vi "TestBed.vi"() -> ()   [LabVIEW 2017]
uses:
  <vilib>/gpm_packages/@cs/Network-sink/Source/Network Interface/Network Interface/Network Interface.lvclass
  f39cf365-6f17-4216-9592-3f82a383dcb0.vi
  <vilib>/gpm_packages/@cs/Network-sink/Source/HeaderMessageProtocol/HeaderMessageProtocol.lvclass
  <vilib>/gpm_packages/@cs/event-logger/Source/String Control Sink/String Control Sink.lvclass
  <vilib>/gpm_packages/@cs/event-logger/Source/Composed Log/Types/Log Level.ctl
  <vilib>/gpm_packages/@cs/event-logger/Source/Composed Log/Composed Log.lvlib
  <vilib>/gpm_packages/@cs/event-logger/Source/Composed Log/LoggerReference/LoggerReference.lvclass
  86a66f69-750b-45a4-9a60-f207d6d0df32.vi
  <vilib>/gpm_packages/@cs/Network-sink/Source/Network Interface/IConnectionFactory/IConnectionFactory.lvclass
  <vilib>/gpm_packages/@cs/Network-sink/Source/Network Interface/IMessagingProtocol/IMessagingProtocol.lvclass
panel:
  out "Array":string[](array[string])
  out "String":string
  out "Numeric 2":dbl
  out "Numeric":dbl
  out "error out":errorcluster
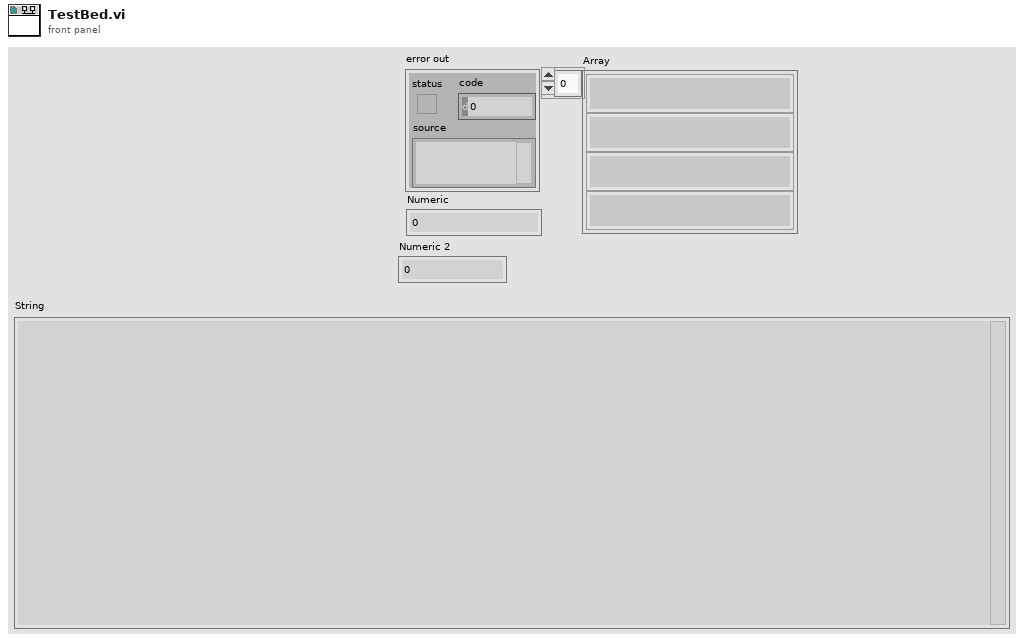
[diagram p1: front panel]
types:
  T1 = typedef "Composed Log.lvlib/Log Level.ctl" = enum16{"Debug", "Info", "Warning", "Error", "Critical"}
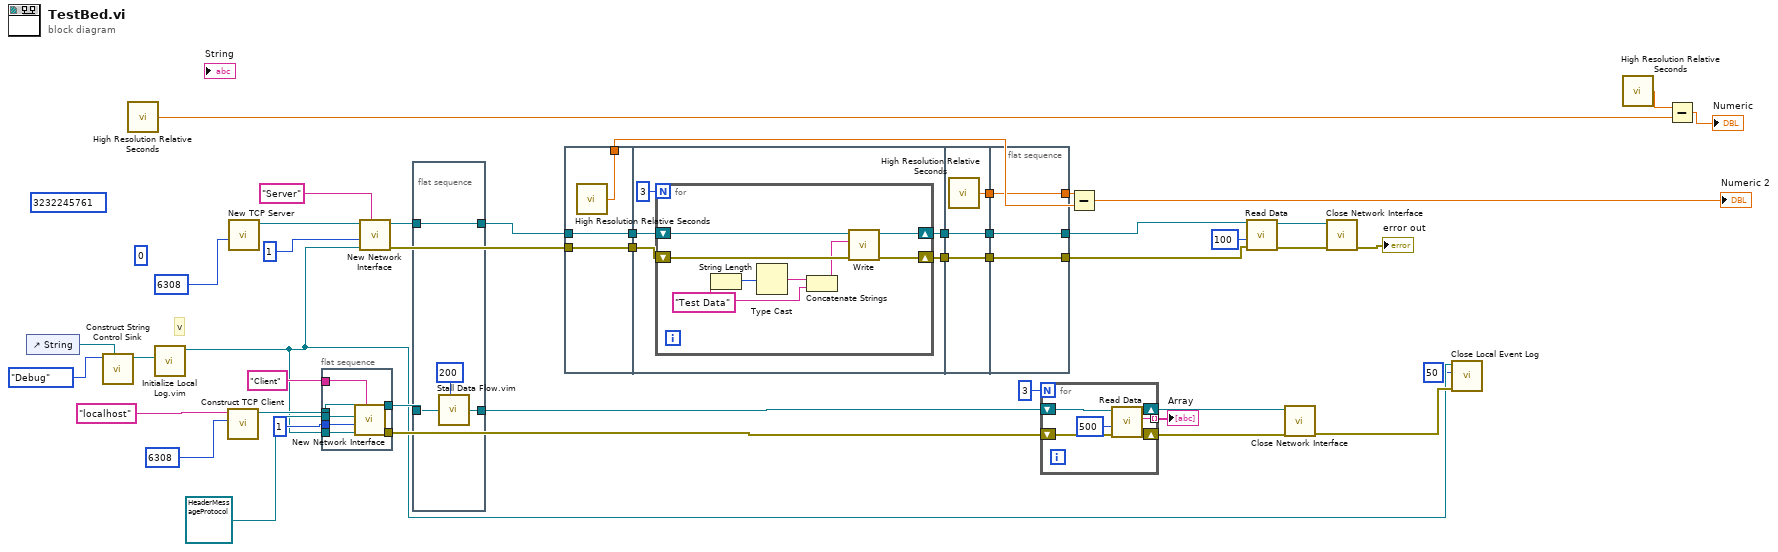
[diagram p0: block diagram]
diagram:
  (unwired) u32 3232245761
  (unwired) u32 0 ("net address")
  # "v"
  n1 = control-ref of="String"() -> (w11:refnum<vi>)
  n2 = call <vilib>:"Construct String Control Sink.vi"("Str Refnum"=w11, "LogLevel"=Log_Level."Debug") -> ("String Control Sink out"=w9:refnum<class "String Control Sink.lvclass">)  [unwired: 9 in]
  n3 = call <vilib>:"High Resolution Relative Seconds.vi"() -> ("relative seconds"=w44:dbl)
  n4 = call "Initialize Local Log.vim"("Startup Sink(s)"=w9) -> ("Log Instance Reference"=w5:refnum<class "LoggerReference.lvclass">)  [unwired: 8 in, 2 out]
  n5 = call <vilib>:"Construct TCP Client.vi"("Remote Port or Service Name"=u16 6308 ("Port"), "Address"="localhost") -> ("TCP Client out"=w39:refnum<class "TCP Client.lvclass">)  [unwired: 9 in]
  n6 = call <vilib>:"New TCP Server.vi"("Port"=u16 6308) -> ("TCP Server out"=w37:refnum<class "TCP Server.lvclass">)  [unwired: 10 in]
  n7 = flat-sequence {
    tunnel: w39 -> [w52]
    tunnel: [w51] -> w29
    tunnel: [w50] -> w24
    tunnel: refnum<class "HeaderMessageProtocol.lvclass"> refnum ("Network Sink.lvlib:HeaderMessageProtocol.lvclass") -> [w49]
    tunnel: 1 ("Max Number of Connections") -> [w48]
    tunnel: "Client" ("Log Alias") -> [w47]
    tunnel: w5 -> [w46]
    frame #0 {
      n8 = call <vilib>:"New Network Interface.vi"("Log Alias"=w47, "Log Instance"=w46, "Max Number of Connections to Create (1)"=w48, "MessageProtocol"=w49, "Connection Factory Type"=w52) -> ("error out"=w51:errorcluster, "Network Interface Reference"=w50:refnum<data-value>)  [unwired: 5 in]
    }
  }
  n9 = call <vilib>:"New Network Interface.vi"("Log Alias"="Server", "Log Instance"=w5, "Max Number of Connections to Create (1)"=1 ("Max Number of Connections"), "Connection Factory Type"=w37) -> ("error out"=w3:errorcluster, "Network Interface Reference"=w25:refnum<data-value>)  [unwired: 6 in]
  n10 = flat-sequence {
    tunnel: [w56] -> w26
    tunnel: w25 -> [w56]
    tunnel: w24 -> [w55]
    tunnel: [w54] -> w23
    frame #0 {
      n11 = call "Stall Data Flow.vim"("value in"=w55, "milliseconds to wait"=u32 200) -> ("value out"=w54:refnum<data-value>)  [unwired: 1 out]
    }
  }
  n12 = flat-sequence {
    tunnel: w26 -> [w58]
    tunnel: w3 -> [w59]
    tunnel: [w59] -> w21
    tunnel: [w58] -> w20
    tunnel: [w57] -> w16
    tunnel: w21 -> [w62]
    tunnel: w20 -> [w61]
    tunnel: [w64] -> w19
    tunnel: [w63] -> w18
    tunnel: w19 -> [w75]
    tunnel: w18 -> [w74]
    tunnel: [w75] -> w14
    tunnel: [w74] -> w13
    tunnel: [w73] -> w12
    tunnel: [w76] -> w17
    tunnel: [w77] -> w42
    tunnel: [w78] -> w43
    tunnel: w14 -> [w78]
    tunnel: w13 -> [w77]
    tunnel: w12 -> [w76]
    frame #0 {
      n13 = call <vilib>:"High Resolution Relative Seconds.vi"() -> ("relative seconds"=w57:dbl)
    }
    frame #1 {
      n14 = for {
        N: 3 -> [_]
        shift-right: [w72] -> w64
        shift-left: w62 -> [w70]
        shift-right: [w71] -> w63
        shift-left: w61 -> [w69]
        w66 = "Test Data" ("Data To Write")
        n15 = String Length(string=w66) -> (length=w68:i32)
        n16 = Type Cast(x=w68) -> (*(type *) &x=w67:string)  [unwired: 1 in]
        n17 = Concatenate Strings(w67, w66) -> (w65:string)
        n18 = call <vilib>:"Write.vi"("error in (no error)"=w70, "Data To Write"=w65, "Network Interface"=w69) -> ("error out"=w72:errorcluster, "Network Interface Out"=w71:refnum<data-value>)  [unwired: 7 in]
      }
    }
    frame #2 {
      n19 = call <vilib>:"High Resolution Relative Seconds.vi"() -> ("relative seconds"=w73:dbl)
    }
    frame #3 {
    }
  }
  n20 = for {
    N: 3 -> [_]
    tunnel: [w80] -> w1 mode=indexing
    shift-right: [w81] -> w27
    shift-left: w29 -> [w84]
    shift-right: [w82] -> w28
    shift-left: w23 -> [w79]
    n21 = call <vilib>:"Read Data.vi"("error in (no error)"=w84, "Timeout in ms (-1)"=500, "Network Interface"=w79) -> ("error out"=w81:errorcluster, "Read Data"=w80:string, "Network Interface Out"=w82:refnum<data-value>)  [unwired: 5 in, 1 out]
  }
  "Array" <- w1
  n22 = Subtract(x=w17, y=w16) -> (x-y=→"Numeric 2":dbl)
  n23 = call <vilib>:"Read Data.vi"("error in (no error)"=w43, "Timeout in ms (-1)"=100, "Network Interface"=w42) -> ("error out"=w34:errorcluster, "Network Interface Out"=w35:refnum<data-value>)  [unwired: 5 in, 2 out]
  n24 = call <vilib>:"Close Network Interface.vi"("error in (no error)"=w27, "Network Interface"=w28) -> ("error out"=w6:errorcluster)  [unwired: 9 in]
  n25 = call <vilib>:"Close Network Interface.vi"("error in (no error)"=w34, "Network Interface"=w35) -> ("error out"=→"error out":errorcluster)  [unwired: 9 in]
  n26 = call <vilib>:"Close Local Event Log.vi"("error in (no error)"=w6, "Deferred Close Time (0 ms)"=u32 50, "Log Instance"=w5) -> ()  [unwired: 8 in, 1 out]
  n27 = call <vilib>:"High Resolution Relative Seconds.vi"() -> ("relative seconds"=w31:dbl)
  n28 = Subtract(x=w31, y=w44) -> (x-y=→"Numeric":dbl)
